vi "客户端.vi"() -> ()   [LabVIEW 2020]
panel:
  in  "停止":bool
  in  "发送按钮":bool
  out "接收信息":string
  in  "发送信息":string
  in  "端口":u16
  in  "IP":string
  out "连接指示灯":bool
  in  "连接按钮":bool
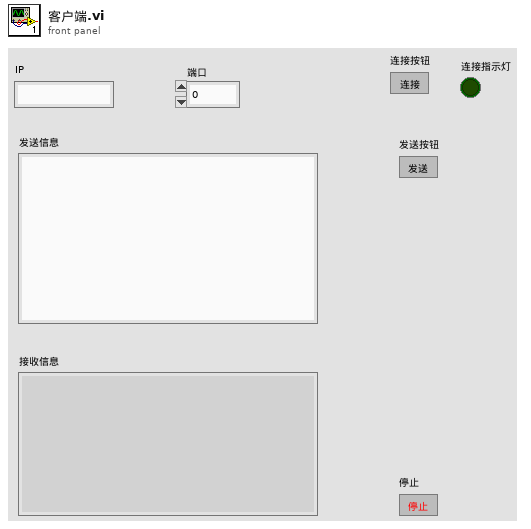
[diagram p1: front panel]
types:
  T1 = enum16{"Standard", "Buffered", "CRLF", "Immediate"}
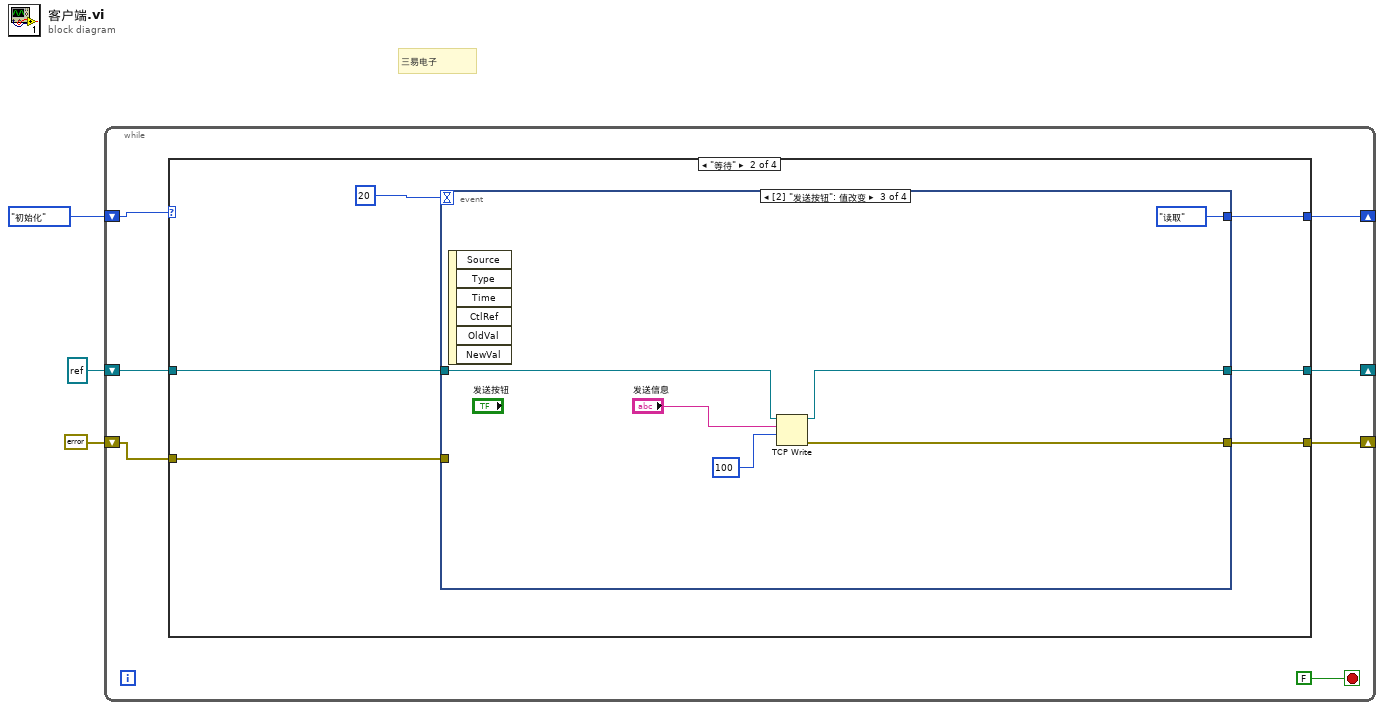
[diagram p0: block diagram]
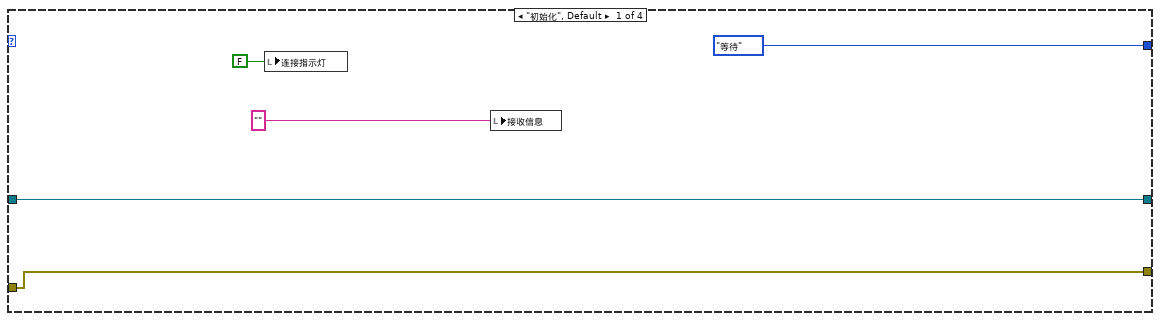
[diagram p2: hidden frame]
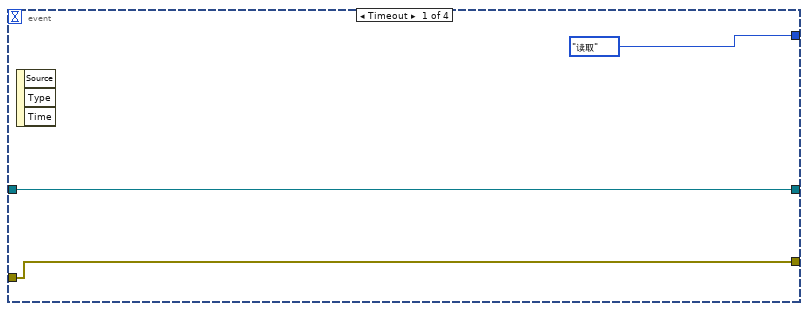
[diagram p3: hidden frame]
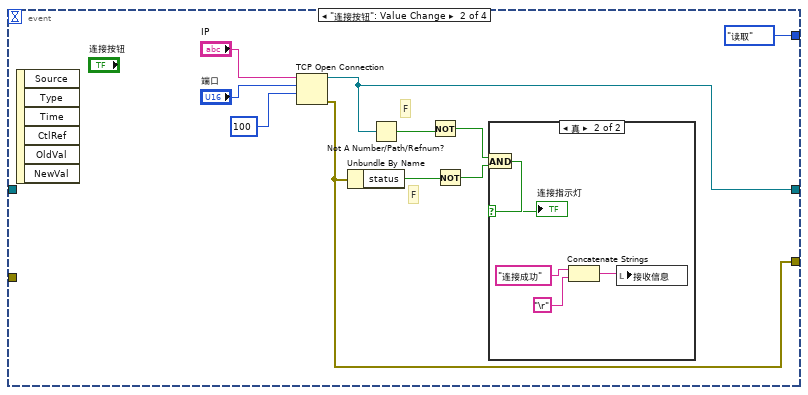
[diagram p4: hidden frame]
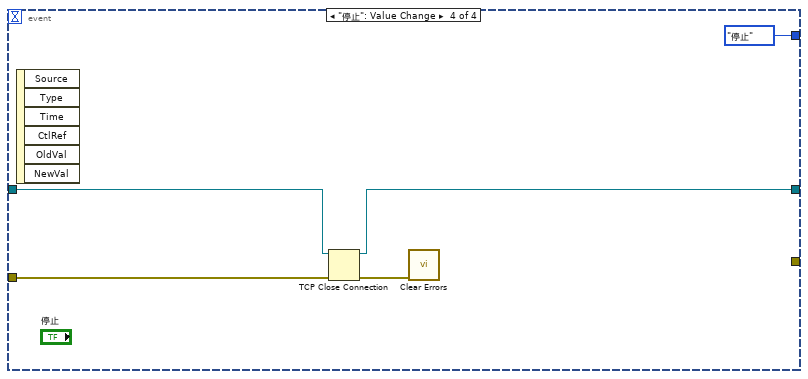
[diagram p6: hidden frame]
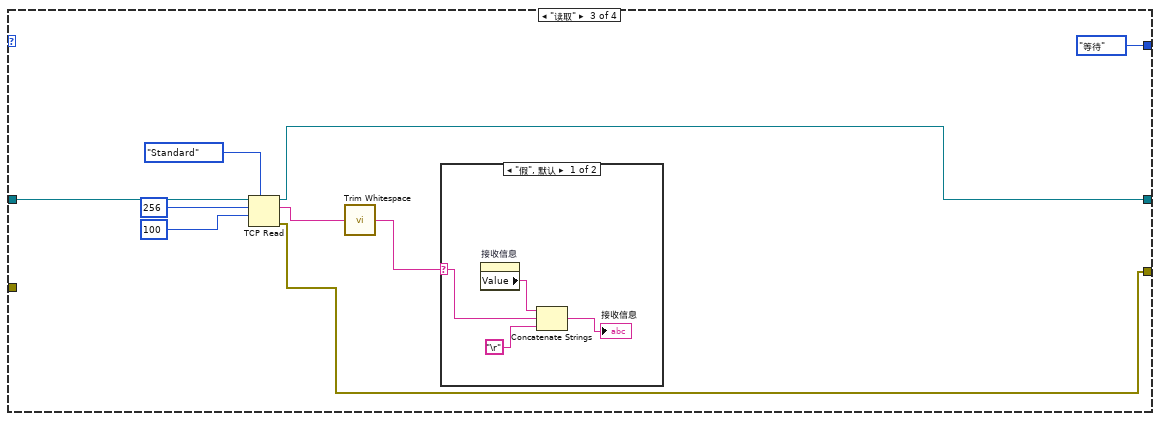
[diagram p7: hidden frame]
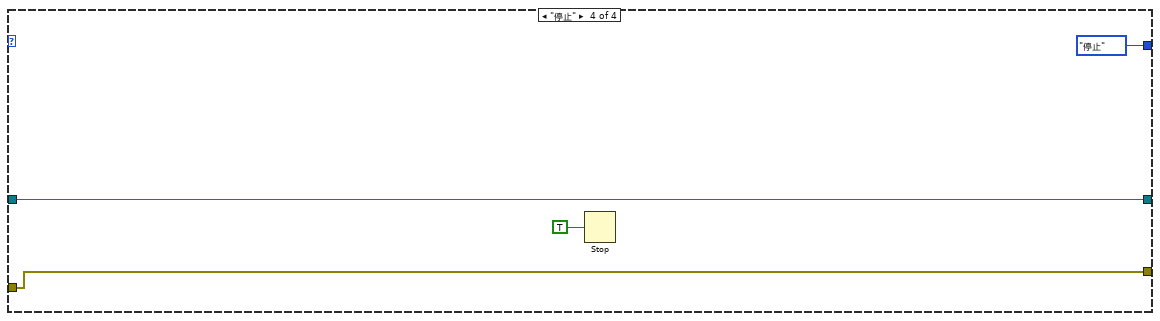
[diagram p9: hidden frame]
diagram:
  # "三易电子"
  n1 = while {
    shift-right: [w8] -> _
    shift-left: enum16{"初始化", "等待", "读取", "停止"}."初始化" -> [w9]
    shift-right: [w7] -> _
    shift-left: refnum<k5> refnum ("connection ID") -> [w6]
    shift-right: [w5] -> _
    shift-left: errorcluster {"status"=FALSE, "code"=0, "source"=""} ("error out") -> [w4]
    stop <- FALSE stop-if-true
    n2 = case shown="\"等待\"" w9 {
      tunnel: [enum16{"初始化", "等待", "读取", "停止"}."等待" w20 enum16{"初始化", "等待", "读取", "停止"}."等待" enum16{"初始化", "等待", "读取", "停止"}."停止"] -> w8
      tunnel: [w12 w19 w55 w65] -> w7
      tunnel: w6 -> [w12 w18 w59 w65]
      tunnel: [w11 w17 w52 w64] -> w5
      tunnel: w4 -> [w11 w16 _ w64]
      frame "初始化", Default {
        n3 = local write "连接指示灯"(FALSE ("连接指示灯")) -> ()
        n4 = local write "接收信息"("" ("接收信息")) -> ()
      }
      frame "等待" {
        n5 = event shown="[2] \"发送按钮\": 值改变" {
          selector: _ -> [_ _ _ _]
          dyn-events: _ -> [_ _ _ _]
          timeout: 20 -> [_ _ _ _]
          tunnel: [enum16{"初始化", "等待", "读取", "停止"}."读取" enum16{"初始化", "等待", "读取", "停止"}."读取" enum16{"初始化", "等待", "读取", "停止"}."读取" enum16{"初始化", "等待", "读取", "停止"}."停止"] -> w20
          tunnel: [w23 w32 w41 w48] -> w19
          tunnel: w18 -> [w23 _ w45 w47]
          tunnel: [w22 w25 w42 _] -> w17
          tunnel: w16 -> [w22 _ _ w50]
          event Timeout {
            n6 = event-data() -> ()  [unwired: 1 in, 3 out]
          }
          event "连接按钮": Value Change {
            # "F"
            # "F"
            n7 = event-data() -> ()  [unwired: 1 in, 6 out]
            n8 = TCP Open Connection(address="IP", remote port or service name="端口", timeout ms (60000)=100 ("超时毫秒(60000)")) -> (connection ID=w32:refnum<k5>, error out=w25:errorcluster)  [unwired: 2 in]
            n9 = Unbundle By Name(w25) -> ("status"=w30:bool)
            n10 = Not A Number/Path/Refnum?(number/path/refnum=w32) -> (NaN/Path/Refnum?=w29:bool)
            n11 = Not(x=w29) -> (.not. x?=w28:bool)
            n12 = Not(x=w30) -> (.not. x?=w27:bool)
            n13 = And(x=w28, y=w27) -> (x .and. y?=w31:bool)
            n14 = case shown="真" w31 {
              selector: w31 -> [_ w39]
              frame False {
              }
              frame True {
                n15 = Concatenate Strings("连接成功" ("接收信息"), "\r") -> (w37:string)
                n16 = local write "接收信息"(w37) -> ()
                "连接指示灯" <- w39
              }
            }
          }
          event "发送按钮": Value Change {
            n17 = event-data() -> ()  [unwired: 1 in, 6 out]
            n18 = TCP Write(connection ID=w45, data in="发送信息", 9:100 ("超时毫秒(25000)")) -> (connection ID out=w41:refnum<k5>, error out=w42:errorcluster)  [unwired: 1 in, 1 out]
          }
          event "停止": Value Change {
            n19 = event-data() -> ()  [unwired: 1 in, 6 out]
            n20 = TCP Close Connection(connection ID=w47, error in (no error)=w50) -> (connection ID out=w48:refnum<k5>, error out=w49:errorcluster)  [unwired: 1 in]
            n21 = call <vilib>:"Clear Errors.vi"("error in (no error)"=w49) -> ()  [unwired: 5 in, 2 out]
          }
        }
      }
      frame "读取" {
        n22 = TCP Read(connection ID=w59, bytes to read=256 ("读取的字节"), 7:T1."Standard" ("模式（标准）"), 9:100 ("超时毫秒(25000)")) -> (connection ID out=w55:refnum<k5>, data out=w54:string, error out=w52:errorcluster)  [unwired: 1 in]
        n23 = call <vilib>:"Trim Whitespace.vi"("string"=w54) -> ("trimmed string"=w53:string)  [unwired: 1 in]
        n24 = case shown="\"假\", 默认" w53 {
          selector: w53 -> [w61 _]
          frame "假", Default {
            n25 = property on="接收信息" class="Str"() -> ("Value"=w62:string)  [unwired: 2 in, 2 out]
            n26 = Concatenate Strings(w62, w61, "\r") -> (→"接收信息":string)
          }
          frame "" {
          }
        }
      }
      frame "停止" {
        n27 = Stop(stop? (T)=TRUE ("停止？(T)")) -> ()
      }
    }
  }
